vi "Init.vi"(8 "error in":errorcluster, 11 "CFG Base in":refnum<class "Red-y Pressure Control CFG Simulated.lvclass">) -> (0 "error out":errorcluster, 3 "CFG Base out":refnum<class "Red-y Pressure Control CFG Simulated.lvclass">)   [LabVIEW 2023, in "Red-y Pressure Control CFG Simulated.lvclass"]
uses:
  Red-y Pressure Control CFG Simulated.lvclass
  D:/git/HAL/HAL GOOP4/Configuration/Configuration JSON/Configuration JSON Base/CFG JSON.lvclass
  Configuration/Configuration JSON/Configuration JSON Base/CFG JSON.lvclass/CFG JSON.ctl
  Pressure Control CFG/Red-y Pressure Control CFG.lvclass
  Red-y Pressure Control CFG Simulated.lvclass/Red-y Pressure Control CFG Simulated.ctl
  Configuration/Configuration JSON/Configuration JSON Base/CFG JSON.lvclass
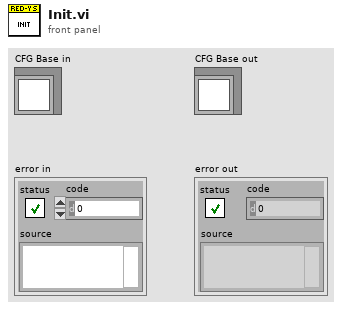
[diagram p1: front panel]
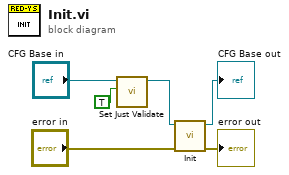
[diagram p0: block diagram]
diagram:
  n1 = call "Set Just Validate.vi"("Just Validate"=TRUE, "CFG JSON Base in"="CFG Base in") -> ("CFG JSON Base out"=w2:refnum<class "Red-y Pressure Control CFG Simulated.lvclass">)  [unwired: 9 in]
  n2 = call-parent "Init.vi"("error in"="error in", "CFG Base in"=w2) -> ("error out"=→"error out":errorcluster, "CFG Base out"=→"CFG Base out":refnum<class "Red-y Pressure Control CFG Simulated.lvclass">)  [unwired: 8 in]
